vi "FTW-Scheduler-Current.vi"(1 "FTW Job Scheduler":refnum<class "FTW-Scheduler.lvclass">) -> (0 "Current Job":string)   [LabVIEW 2014, in "FTW-Scheduler.lvclass"]
uses:
  FTW-Scheduler.lvclass
  FTW-Scheduler.lvclass/FTW-Scheduler.ctl
panel:
  # "Inputs"
  # "Outputs"
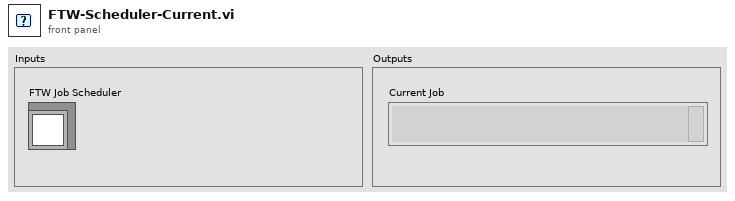
[diagram p1: front panel]
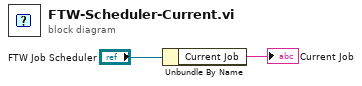
[diagram p0: block diagram]
diagram:
  n1 = Unbundle By Name("FTW Job Scheduler") -> ("Current Job"=→"Current Job":string)
